vi "Authenticate.vi"(8 "error in (no error)":errorcluster, 9 "Password":string, 10 "Username":string, 11 "I Authentication Provider in":refnum<class "I Authentication Provider.lvclass">) -> (0 "error out":errorcluster, 2 "User":refnum<class "User.lvclass">, 3 "I Authentication Provider out":refnum<class "I Authentication Provider.lvclass">)   [LabVIEW 2026, in "I Authentication Provider.lvclass"]
uses:
  I Authentication Provider.lvclass
  Domain/User/User.lvclass
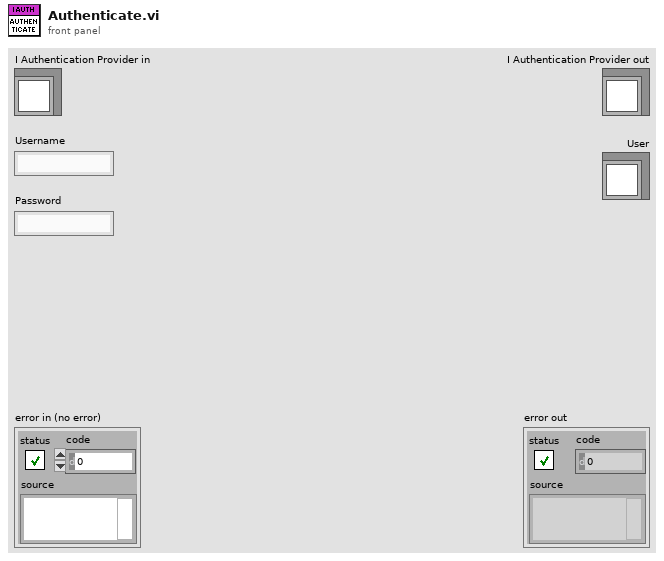
[diagram p1: front panel]
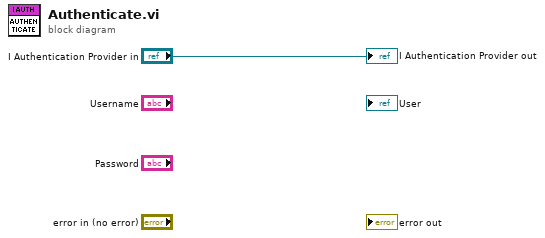
[diagram p0: block diagram]
diagram:
  "I Authentication Provider out" <- "I Authentication Provider in"
